vi "STFT - Spectogram.vi"(0 "reference in":refnum<class "SPWB.lvclass">, 5 "error in (no error)":errorcluster, 7 "Ch. Idx":i32, 9 "STFT Parameters":T1={"SVM time segment"={"from [s]"=-1.0, "to [s]"=-1.0, "time increment"=100.0, "time increment units (%)"=enum."%"}, "FFT block size"=1024, "Window type"=1, "dB On (T)"=FALSE, "weighting"=0, "Norm Signal"=FALSE, "time steps"=-1, "STFT Type"=enum."TFA Pkg - STFT", "Color Table"=enum."rainbow"} {"weighting" items=["Linear", "A-weighting", "B-weighting", "C-weighting"]; "Window type" items=["None ", "Hanning", "Hamming", "Blackman-Harris", "Exact Blackman", "Blackman", "Flat Top", "4 Term B-Harris ", "7 Term B-Harris", "Low Sidelobe", "Gaussian"]; "FFT block size" min=1; "SVM time segment"."time increment" format="%.2f"; "SVM time segment"."to [s]" format="%.2f"; "SVM time segment"."from [s]" format="%.2f"}) -> (11 "scale info":variant, 12 "spectrogram UI":dbl[][](array[numeric]), 13 "spectrogram Trends":dbl[][](array[numeric]), 14 "reference out":refnum<class "SPWB.lvclass">, 19 "error out":errorcluster)   [LabVIEW 2020, in "SPWB.lvclass"]
uses:
  SPWB.lvclass
  <vilib>/addons/Time Series Analysis/Series Preprocess.llb/TSA Resampling (Waveform).vi
  <vilib>/addons/Time Frequency Analysis/Spectrogram.llb/TFA STFT Spectrogram (Waveform).vi
  API/GSwFormDSP_class/GSwFormDSP.lvclass
  <vilib>/addons/_Advanced Signal Processing/NI_AdvSigProcTSA.lvlib
  <vilib>/addons/_Advanced Signal Processing/NI_AdvSigProcTFA.lvlib
panel:
  out "Nb Time Steps":i32
  out "Nb Freq.":i32
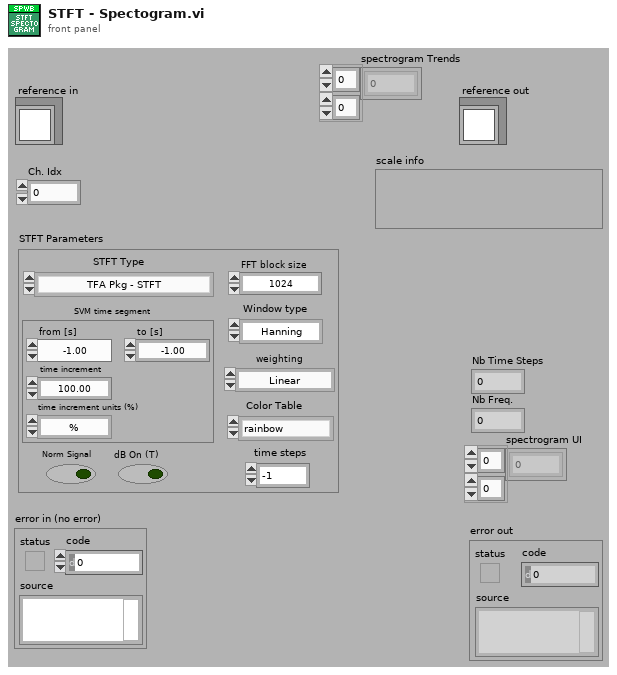
[diagram p1: front panel]
types:
  T1 = cluster{"SVM time segment":cluster{"from [s]":dbl, "to [s]":dbl, "time increment":dbl, "time increment units (%)":enum16{"%", "s", "ms"}}, "FFT block size":i32, "Window type":i32, "dB On (T)":bool, "weighting":u16, "Norm Signal":bool, "time steps":i32, "STFT Type":enum16{"SVM -STFT", "TFA Pkg - STFT"}, "Color Table":enum16{"fire", "rainbow", "grey", "inverse grey", "ice", "original"}}
  T2 = enum16{"None", "To itself", "To the max levels of ALL the signals"}
  T3 = typedef "SPWB.lvclass/ObjectAttributes.ctl" = cluster{"Window Name Index":string, "Data":refnum<class "GSwFormDSP.lvclass">, "Registration":refnum<class "Registration.lvclass">, "TFA User Control Refs ":T4}
  T4 = typedef "SPWB.lvclass/TFA - User Control References.ctl" = cluster{"STFT Graph":refnum<vi>, "Time Section":refnum<vi>, "Frequency Section":refnum<vi>}
  T5 = enum16{"fire", "rainbow", "grey", "inverse grey", "ice", "original"}
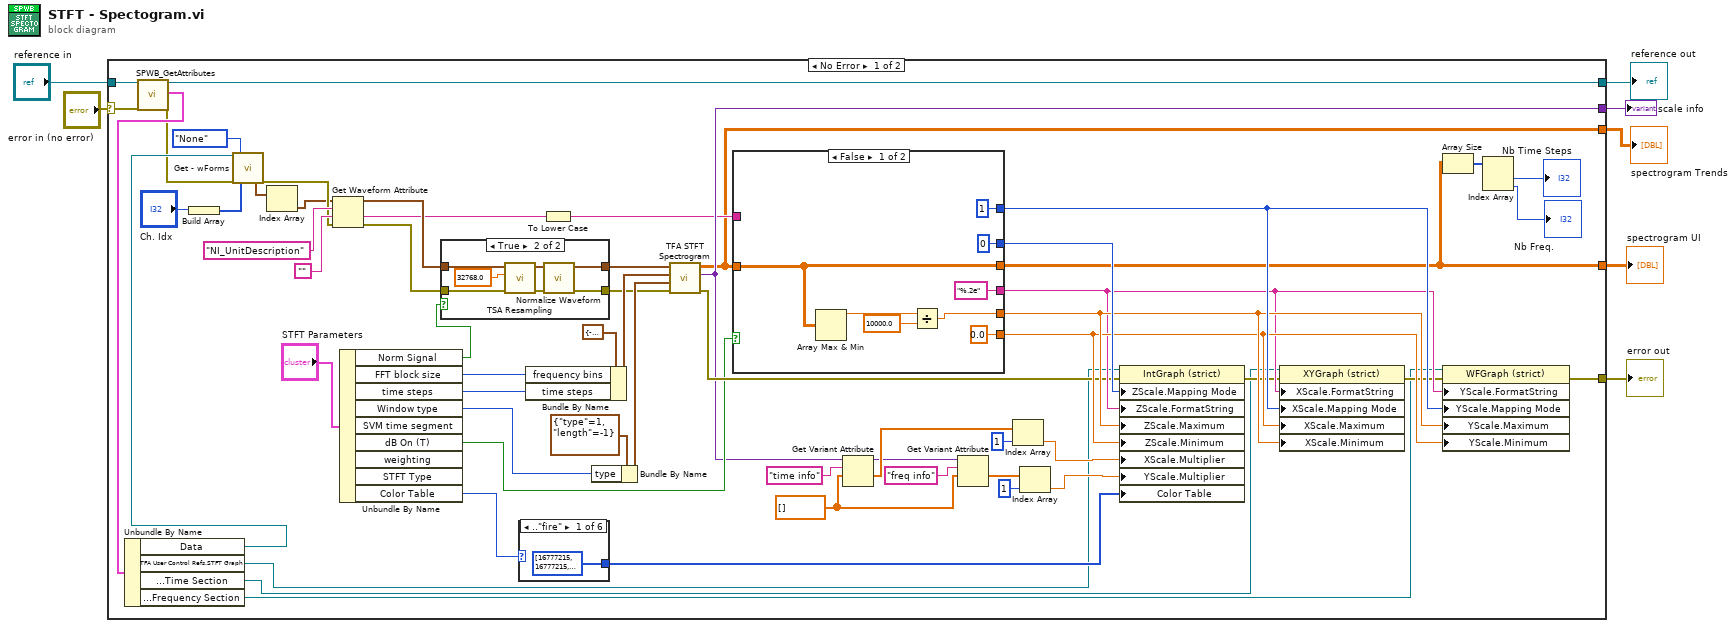
[diagram p0: block diagram]
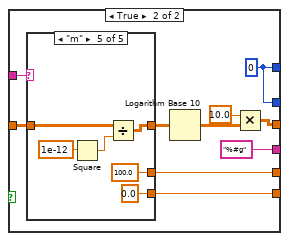
[diagram p2: hidden frame]
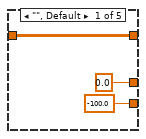
[diagram p3: hidden frame]
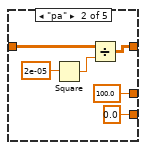
[diagram p4: hidden frame]
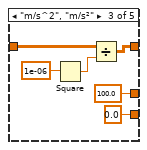
[diagram p5: hidden frame]
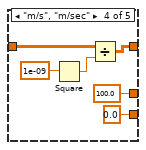
[diagram p6: hidden frame]
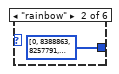
[diagram p7: hidden frame]
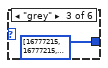
[diagram p8: hidden frame]
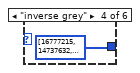
[diagram p9: hidden frame]
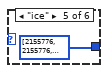
[diagram p10: hidden frame]
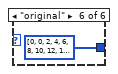
[diagram p11: hidden frame]
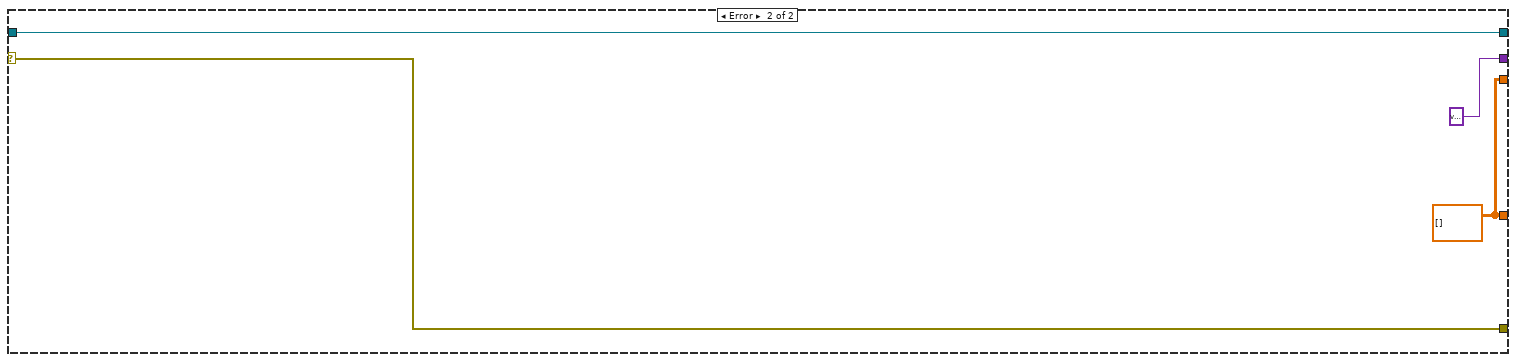
[diagram p13: hidden frame]
diagram:
  n1 = case shown="No Error" "error in (no error)" {
    selector: "error in (no error)" -> [w67 w131]
    tunnel: [w27 w131] -> w6
    tunnel: [w66 w130] -> w4
    tunnel: "reference in" -> [w65 w130]
    tunnel: [w26 w128] -> w3
    tunnel: [w25 variant ("scale info")] -> w2
    tunnel: [w18 w128] -> w1
    frame No Error {
      w58 = dbl[] []
      n2 = call "SPWB_GetAttributes.vi"("reference in"=w65, "error in (no error)"=w67) -> ("reference out"=w66:refnum<class "SPWB.lvclass">, "attributes"=w32:T3, "error out"=w15:errorcluster)  [unwired: 14 in, 1 out]
      n3 = Unbundle By Name(w32) -> ("Data"=w17:refnum<class "GSwFormDSP.lvclass">, "TFA User Control Refs.STFT Graph"=w31:refnum<vi>, "TFA User Control Refs.Time Section"=w30:refnum<vi>, "TFA User Control Refs.Frequency Section"=w29:refnum<vi>)
      n4 = Build Array("Ch. Idx") -> (w13:i32[])
      n5 = call-dynamic "Get - wForms.vi"("reference in"=w17, "error in (no error)"=w15, "Normalization Option"=T2."None", "Indexes (Empty = ALL)"=w13) -> ("wForms"=w11:waveform(dbl)[], "error out"=w12:errorcluster)  [unwired: 12 in, 2 out]
      n6 = Index Array(array=w11) -> (element=w10:waveform(dbl))  [unwired: 1 in]
      n7 = Get Waveform Attribute(4:w12, 5:"", 6:"NI_UnitDescription" ("Att - wform unit"), 7:w10) -> (0:w23:errorcluster, 1:w20:string, 3:w24:waveform(dbl))  [unwired: 1 out]
      n8 = Unbundle By Name("STFT Parameters") -> ("Norm Signal"=w38:bool, "FFT block size"=w9:i32, "time steps"=w8:i32, "Window type"=w34:i32, "dB On (T)"=w33:bool, "Color Table"=w37:T5)  [unwired: 3 out]
      n9 = case shown="True" w38 {
        tunnel: [w120 w127] -> w35
        tunnel: w24 -> [w120 w126]
        tunnel: w23 -> [w119 w122]
        tunnel: [w119 w121] -> w36
        frame False {
        }
        frame True {
          n10 = call-poly <vilib>:"TSA Resampling.vi"("error in (no error)"=w122, "new sampling rate"=32768.0, "Xt"=w126) -> ("error out"=w123:errorcluster, "Xt resampled"=w124:waveform(dbl))  [unwired: 7 in]
          n11 = call <vilib>:"Normalize Waveform.vi"("error in (no error)"=w123, "waveform in"=w124) -> ("error out"=w121:errorcluster, "normalized waveform"=w127:waveform(dbl))  [unwired: 6 in, 2 out]
        }
      }
      n12 = case shown="..\"fire\"" w37 {
        tunnel: [u32[] [16777215, 16777215, 16777215, 16777215, 16777215, 16777215, 16777215, 16777215, 16777212, 16777209, 16777205, 16777202, 16777199, 16777196, 16777193, 16777190, 16777186, 16777183, 16777180, 16777177, 16777174, 16777170, 16777167, 16777164, 16777161, 16777158, 16777154, 16777151, 16777148, 16777145, 16777142, 16777139, 16777135, 16777132, 16777129, 16777126, 16777123, 16777119, 16777116, 16777113, 16777110, 16777107, 16777103, 16777100, 16777097, 16777094, 16777091, 16777088, 16777084, 16777081, 16777078, 16777075, 16777072, 16777068, 16777065, 16777062, 16777059, 16777056, 16777052, 16777049, 16777046, 16777043, 16777040, 16777037, 16777033, 16777030, 16777027, 16777024, 16777021, 16777017, 16777014, 16777011, 16777008, 16777005, 16777001, 16776998, 16776995, 16776992, 16776989, 16776986, 16776982, 16776979, 16776976, 16776973, 16776970, 16776966, 16776963, 16776960, 16776192, 16775424, 16774400, 16773632, 16772864, 16772096, 16771328, 16770560, 16769536, 16768768, 16768000, 16767232, 16766464, 16765440, 16764672, 16763904, 16763136, 16762368, 16761344, 16760576, 16759808, 16759040, 16758272, 16757504, 16756480, 16755712, 16754944, 16754176, 16753408, 16752384, 16751616, 16750848, 16750080, 16749312, 16748288, 16747520, 16746752, 16745984, 16745216, 16744448, 16743424, 16742656, 16741888, 16741120, 16740352, 16739328, 16738560, 16737792, 16737024, 16736256, 16735232, 16734464, 16733696, 16732928, 16732160, 16731392, 16730368, 16729600, 16728832, 16728064, 16727296, 16726272, 16725504, 16724736, 16723968, 16723200, 16722176, 16721408, 16720640, 16719872, 16719104, 16718336, 16717312, 16716544, 16715776, 16715008, 16714240, 16713216, 16712448, 16711680, 16515072, 16318464, 16056320, 15859712, 15663104, 15466496, 15269888, 15073280, 14811136, 14614528, 14417920, 14221312, 14024704, 13762560, 13565952, 13369344, 13172736, 12976128, 12713984, 12517376, 12320768, 12124160, 11927552, 11730944, 11468800, 11272192, 11075584, 10878976, 10682368, 10420224, 10223616, 10027008, 9830400, 9633792, 9371648, 9175040, 8978432, 8781824, 8585216, 8388608, 8126464, 7929856, 7733248, 7536640, 7340032, 7077888, 6881280, 6684672, 6488064, 6291456, 6029312, 5832704, 5636096, 5439488, 5242880, 5046272, 4784128, 4587520, 4390912, 4194304, 3997696, 3735552, 3538944, 3342336, 3145728, 2949120, 2686976, 2490368, 2293760, 2097152, 1900544, 1703936, 1441792, 1245184, 1048576, 851968, 655360, 393216, 196608, 65793, 65793, 65793, 65793, 65793, 65793, 65793, 65793, 0] ("256 fire") u32[] [0, 8388863, 8257791, 8061183, 7930111, 7733503, 7602431, 7405823, 7274751, 7078143, 6947071, 6750463, 6619391, 6422783, 6291711, 6095103, 5964031, 5767423, 5636351, 5439743, 5308671, 5112063, 4980991, 4784383, 4653311, 4456703, 4325631, 4129023, 3932415, 3801343, 3604735, 3473663, 3277055, 3145983, 2949375, 2818303, 2621695, 2490623, 2294015, 2162943, 1966335, 1835263, 1638655, 1507583, 1310975, 1179903, 983295, 852223, 655615, 524543, 327935, 196863, 511, 1791, 3071, 4351, 5631, 6911, 8191, 9471, 10751, 12031, 13311, 14591, 15871, 17151, 18431, 19711, 20991, 22271, 23551, 24831, 26111, 27391, 28671, 29951, 31231, 32511, 33791, 35071, 36351, 37631, 38911, 40191, 41471, 42751, 44031, 45311, 46591, 47871, 49151, 50431, 51711, 52991, 54271, 55551, 56831, 58111, 59391, 60671, 61951, 63231, 64511, 65532, 65527, 65522, 65517, 65512, 65507, 65502, 65497, 65492, 65487, 65482, 65477, 65472, 65467, 65462, 65457, 65452, 65447, 65442, 65437, 65432, 65427, 65422, 65417, 65412, 65407, 65402, 65397, 65392, 65387, 65382, 65377, 65372, 65367, 65362, 65357, 65352, 65347, 65342, 65337, 65332, 65327, 65322, 65317, 65312, 65307, 65302, 65297, 65292, 65287, 65282, 261888, 589568, 917248, 1244928, 1572608, 1900288, 2227968, 2555648, 2883328, 3211008, 3538688, 3866368, 4194048, 4521728, 4849408, 5177088, 5504768, 5832448, 6160128, 6487808, 6815488, 7143168, 7470848, 7798528, 8126208, 8453888, 8781568, 9109248, 9436928, 9764608, 10092288, 10419968, 10747648, 11075328, 11403008, 11730688, 12058368, 12386048, 12713728, 13041408, 13369088, 13696768, 14024448, 14352128, 14679808, 15007488, 15335168, 15662848, 15990528, 16318208, 16645888, 16775936, 16774656, 16773376, 16772096, 16770816, 16769536, 16768256, 16766976, 16765696, 16764416, 16763136, 16761856, 16760576, 16759296, 16758016, 16756736, 16755456, 16754176, 16752896, 16751616, 16750336, 16749056, 16747776, 16746496, 16745216, 16743936, 16742656, 16741376, 16740096, 16738816, 16737536, 16736256, 16734976, 16733696, 16732416, 16731136, 16729856, 16728576, 16727296, 16726016, 16724736, 16723456, 16722176, 16720896, 16719616, 16718336, 16717056, 16715776, 16714496, 16713216, 16711680] ("rainbow") u32[] [16777215, 16777215, 16777215, 16777215, 16777215, 16777215, 16711422, 16711422, 16711422, 16711422, 16711422, 16645629, 16645629, 16645629, 16645629, 16645629, 16645629, 16579836, 16579836, 16579836, 16579836, 16579836, 16514043, 16514043, 16514043, 16514043, 16514043, 16448250, 16448250, 16448250, 16448250, 16448250, 16316664, 16382457, 16382457, 16382457, 16382457, 16316664, 16316664, 16316664, 16316664, 16250871, 16250871, 16250871, 16250871, 16250871, 16185078, 16185078, 16185078, 16185078, 16119285, 16119285, 16119285, 16119285, 16119285, 16053492, 16053492, 16053492, 16053492, 15987699, 15987699, 15987699, 15987699, 15921906, 15987699, 15921906, 15921906, 15856113, 15856113, 15856113, 15856113, 15856113, 15790320, 15790320, 15790320, 15724527, 15724527, 15724527, 15724527, 15658734, 15658734, 15658734, 15658734, 15592941, 15592941, 15592941, 15592941, 15527148, 15527148, 15527148, 15461355, 15461355, 15461355, 15461355, 15395562, 15395562, 15395562, 15395562, 15329769, 15329769, 15329769, 15263976, 15263976, 15263976, 15198183, 15198183, 15198183, 15198183, 15132390, 15132390, 15132390, 15066597, 15066597, 15066597, 15000804, 15000804, 15000804, 14935011, 14935011, 14935011, 14869218, 14869218, 14869218, 14803425, 14803425, 14803425, 14737632, 14737632, 14671839, 14671839, 14671839, 14606046, 14606046, 14606046, 14540253, 14540253, 14540253, 14474460, 14474460, 14408667, 14408667, 14408667, 14342874, 14342874, 14277081, 14277081, 14277081, 14211288, 14211288, 14145495, 14145495, 14079702, 14079702, 14013909, 14013909, 14013909, 13948116, 13948116, 13882323, 13882323, 13816530, 13816530, 13750737, 13750737, 13684944, 13684944, 13619151, 13619151, 13553358, 13553358, 13487565, 13487565, 13421772, 13421772, 13355979, 13290186, 13290186, 13224393, 13224393, 13158600, 13092807, 13092807, 13027014, 13027014, 12961221, 12895428, 12895428, 12829635, 12763842, 12763842, 12698049, 12632256, 12566463, 12566463, 12500670, 12434877, 12434877, 12369084, 12303291, 12237498, 12171705, 12171705, 12105912, 12040119, 11974326, 11908533, 11842740, 11776947, 11711154, 11645361, 11579568, 11513775, 11447982, 11382189, 11316396, 11250603, 11184810, 11119017, 10987431, 10921638, 10855845, 10790052, 10658466, 10592673, 10461087, 10395294, 10329501, 10197915, 10066329, 10000536, 9868950, 9737364, 9605778, 9474192, 9342606, 9211020, 9079434, 8882055, 8750469, 8553090, 8421504, 8224125, 7960953, 7763574, 7500402, 7237230, 6974058, 6645093, 6316128, 5855577, 5395026, 4868682, 4210752, 3289650, 2105376, 0] ("256 log up") u32[] [16777215, 14737632, 13487565, 12632256, 11908533, 11382189, 10921638, 10526880, 10132122, 9803157, 9539985, 9276813, 9013641, 8816262, 8553090, 8421504, 8224125, 8026746, 7895160, 7697781, 7566195, 7434609, 7303023, 7171437, 7039851, 6908265, 6776679, 6710886, 6579300, 6447714, 6381921, 6316128, 6184542, 6118749, 5987163, 5921370, 5855577, 5789784, 5658198, 5592405, 5526612, 5460819, 5395026, 5329233, 5263440, 5197647, 5131854, 5066061, 5000268, 4934475, 4868682, 4802889, 4737096, 4671303, 4605510, 4605510, 4539717, 4473924, 4408131, 4342338, 4342338, 4276545, 4210752, 4210752, 4144959, 4079166, 4013373, 4013373, 3947580, 3881787, 3881787, 3815994, 3750201, 3750201, 3684408, 3684408, 3618615, 3552822, 3552822, 3487029, 3487029, 3421236, 3421236, 3355443, 3289650, 3289650, 3223857, 3223857, 3158064, 3158064, 3092271, 3092271, 3026478, 3026478, 2960685, 2960685, 2894892, 2894892, 2829099, 2829099, 2763306, 2763306, 2763306, 2697513, 2697513, 2631720, 2631720, 2565927, 2565927, 2500134, 2500134, 2500134, 2434341, 2434341, 2368548, 2368548, 2368548, 2302755, 2302755, 2236962, 2236962, 2236962, 2171169, 2171169, 2171169, 2105376, 2105376, 2105376, 2039583, 2039583, 1973790, 1973790, 1973790, 1907997, 1907997, 1907997, 1842204, 1842204, 1842204, 1776411, 1776411, 1776411, 1710618, 1710618, 1710618, 1644825, 1644825, 1644825, 1579032, 1579032, 1579032, 1579032, 1513239, 1513239, 1513239, 1447446, 1447446, 1447446, 1381653, 1381653, 1381653, 1381653, 1315860, 1315860, 1315860, 1315860, 1250067, 1250067, 1250067, 1184274, 1184274, 1184274, 1184274, 1118481, 1118481, 1118481, 1118481, 1052688, 1052688, 1052688, 1052688, 986895, 986895, 986895, 921102, 921102, 921102, 921102, 921102, 855309, 855309, 855309, 855309, 789516, 789516, 789516, 789516, 723723, 723723, 723723, 723723, 657930, 657930, 657930, 657930, 657930, 592137, 592137, 592137, 592137, 526344, 526344, 526344, 526344, 526344, 460551, 460551, 460551, 460551, 460551, 394758, 394758, 394758, 394758, 328965, 328965, 328965, 328965, 328965, 263172, 263172, 263172, 263172, 263172, 197379, 197379, 197379, 197379, 197379, 131586, 131586, 131586, 131586, 131586, 131586, 65793, 65793, 65793, 65793, 65793, 0, 0, 0, 0, 0, 0] ("256 log down") u32[] [2155776, 2155776, 2155776, 2155776, 2155776, 2155776, 2155776, 2155776, 127491, 127491, 127491, 127491, 127491, 127491, 127491, 127491, 522752, 522752, 522752, 522752, 522752, 522752, 522752, 522752, 64018, 64018, 64018, 64018, 64018, 64018, 64018, 64018, 63778, 63778, 63778, 63778, 63778, 63778, 63778, 63778, 63790, 63790, 63790, 63790, 63790, 63790, 63790, 63790, 63797, 63797, 63797, 63797, 63797, 63797, 63797, 63797, 63807, 63807, 63807, 63807, 63807, 63807, 63807, 63807, 64068, 64068, 64068, 64068, 64068, 64068, 64068, 64068, 63828, 63828, 63828, 63828, 63828, 63828, 63828, 63828, 63833, 63833, 63833, 63833, 63833, 63833, 63833, 63833, 63836, 63836, 63836, 63836, 63836, 63836, 63836, 63836, 63836, 63836, 63836, 63836, 63836, 63836, 63836, 63836, 61790, 61790, 61790, 61790, 61790, 61790, 61790, 61790, 58464, 58464, 58464, 58464, 58464, 58464, 58464, 58464, 55387, 55387, 55387, 55387, 55387, 55387, 55387, 55387, 51286, 51286, 51286, 51286, 51286, 51286, 51286, 51286, 47440, 47440, 47440, 47440, 47440, 47440, 47440, 47440, 40284, 40284, 40284, 40284, 40284, 40284, 40284, 40284, 34154, 34154, 34154, 34154, 34154, 34154, 34154, 34154, 28540, 28540, 28540, 28540, 28540, 28540, 28540, 28540, 20113, 20113, 20113, 20113, 20113, 20113, 20113, 20113, 12193, 12193, 12193, 12193, 12193, 12193, 12193, 12193, 12714, 12714, 12714, 12714, 12714, 12714, 12714, 12714, 7351, 7351, 7351, 7351, 7351, 7351, 7351, 7351, 4800, 4800, 4800, 4800, 4800, 4800, 4800, 4800, 195, 195, 195, 195, 195, 195, 195, 195, 189, 189, 189, 189, 189, 189, 189, 189, 183, 183, 183, 183, 183, 183, 183, 183, 175, 175, 175, 175, 175, 175, 175, 175, 164, 164, 164, 164, 164, 164, 164, 164, 155, 155, 155, 155, 155, 155, 155, 155] ("32 ice") u32[] [0, 0, 2, 4, 6, 8, 10, 12, 14, 16, 18, 20, 22, 24, 26, 28, 30, 32, 34, 36, 38, 40, 42, 44, 46, 48, 50, 52, 54, 56, 58, 60, 62, 64, 66, 68, 70, 72, 74, 76, 78, 80, 82, 84, 86, 88, 90, 92, 94, 96, 98, 100, 102, 104, 106, 108, 110, 112, 114, 116, 118, 120, 122, 124, 126, 128, 130, 132, 134, 136, 138, 140, 142, 144, 146, 148, 150, 152, 154, 156, 158, 160, 162, 164, 166, 168, 170, 172, 174, 176, 178, 180, 182, 184, 186, 188, 190, 192, 194, 196, 198, 200, 202, 204, 206, 208, 210, 212, 214, 216, 218, 220, 222, 224, 226, 228, 230, 232, 234, 236, 238, 240, 242, 244, 246, 248, 250, 252, 255, 131839, 263423, 395007, 526591, 658175, 789759, 921343, 1052927, 1184511, 1316095, 1447679, 1579263, 1710847, 1842431, 1974015, 2105599, 2237183, 2368767, 2500351, 2631935, 2763519, 2895103, 3026687, 3158271, 3289855, 3421439, 3553023, 3684607, 3816191, 3947775, 4079359, 4210943, 4342527, 4474111, 4605695, 4737279, 4868863, 5000447, 5132031, 5263615, 5395199, 5526783, 5658367, 5789951, 5921535, 6053119, 6184703, 6316287, 6447871, 6579455, 6711039, 6842623, 6974207, 7105791, 7237375, 7368959, 7500543, 7632127, 7763711, 7895295, 8026879, 8158463, 8290047, 8421631, 8553215, 8684799, 8816383, 8947967, 9079551, 9211135, 9342719, 9474303, 9605887, 9737471, 9869055, 10000639, 10132223, 10263807, 10395391, 10526975, 10658559, 10790143, 10921727, 11053311, 11184895, 11316479, 11448063, 11579647, 11711231, 11842815, 11974399, 12105983, 12237567, 12369151, 12500735, 12632319, 12763903, 12895487, 13027071, 13158655, 13290239, 13421823, 13553407, 13684991, 13816575, 13948159, 14079743, 14211327, 14342911, 14474495, 14606079, 14737663, 14869247, 15000831, 15132415, 15263999, 15395583, 15527167, 15658751, 15790335, 15921919, 16053503, 16185087, 16316671, 16448255, 16579839, 16777215] ("original")] -> w42
        frame .."fire" {
        }
        frame "rainbow" {
        }
        frame "grey" {
        }
        frame "inverse grey" {
        }
        frame "ice" {
        }
        frame "original" {
        }
      }
      n13 = Bundle By Name(cluster=cluster{"time steps":i32, "frequency bins":i32} {"time steps"=-1, "frequency bins"=512} ("time-frequency sampling info"), "frequency bins"=w9, "time steps"=w8) -> (w54:cluster{"time steps":i32, "frequency bins":i32})
      n14 = To Lower Case(string=w20) -> (all lower case string=w19:string)
      n15 = Bundle By Name(cluster=cluster{"type":i32, "length":i32} {"type"=1, "length"=-1} ("window info"), "type"=w34) -> (w63:cluster{"type":i32, "length":i32})
      n16 = call-poly <vilib>:"TFA STFT Spectrogram.vi"("error in (no error)"=w36, "window info"=w63, "time-frequency sampling info"=w54, "signal"=w35) -> ("error out"=w39:errorcluster, "scale info"=w25:variant, "spectrogram"=w18:dbl[][])  [unwired: 5 in]
      n17 = case shown="False" w33 {
        tunnel: w18 -> [w74 w79]
        tunnel: [w74 w83] -> w26
        tunnel: [w71 w78] -> w47
        tunnel: [0.0 w77] -> w46
        tunnel: ["%.2e" "%#g"] -> w45
        tunnel: [u8 1 ("X Scale.Mapping Mode") w82] -> w48
        tunnel: [u8 0 ("X Scale.Mapping Mode") w82] -> w49
        tunnel: w19 -> [_ w81]
        frame False {
          n18 = Array Max & Min(array=w74) -> (max value=w72:dbl)  [unwired: 3 out]
          n19 = Divide(x=w72, y=10000.0) -> (x/y=w71:dbl)
        }
        frame True {
          w82 = u8 0 ("X Scale.Mapping Mode")
          n20 = case shown="\"m\"" w81 {
            tunnel: [w88 w93 w99 w105 w111] -> w80
            tunnel: w79 -> [w88 w94 w100 w106 w112]
            tunnel: [0.0 100.0 100.0 100.0 100.0] -> w78
            tunnel: [-100.0 0.0 0.0 0.0 0.0] -> w77
            frame "", Default {
            }
            frame "pa" {
              n21 = Square(x=2e-05) -> (x^2=w91:dbl)
              n22 = Divide(x=w94, y=w91) -> (x/y=w93:dbl[][])
            }
            frame "m/s^2", "m/s²" {
              n23 = Square(x=1e-06) -> (x^2=w98:dbl)
              n24 = Divide(x=w100, y=w98) -> (x/y=w99:dbl[][])
            }
            frame "m/s", "m/sec" {
              n25 = Square(x=1e-09) -> (x^2=w104:dbl)
              n26 = Divide(x=w106, y=w104) -> (x/y=w105:dbl[][])
            }
            frame "m" {
              n27 = Square(x=1e-12) -> (x^2=w110:dbl)
              n28 = Divide(x=w112, y=w110) -> (x/y=w111:dbl[][])
            }
          }
          n29 = Logarithm Base 10(1:w80) -> (0:w85:dbl[][])
          n30 = Multiply(x=10.0, y=w85) -> (x*y=w83:dbl[][])
        }
      }
      n31 = Get Variant Attribute(Variant=w25, name="time info", default value (empty Variant)=w58) -> (duplicate Variant=w59:variant, value=w61:dbl[])  [unwired: 1 in, 2 out]
      n32 = Get Variant Attribute(Variant=w59, name="freq info", default value (empty Variant)=w58) -> (value=w64:dbl[])  [unwired: 1 in, 3 out]
      n33 = Index Array(array=w61, index=1) -> (element=w40:dbl)
      n34 = Index Array(array=w64, index=1) -> (element=w41:dbl)
      n35 = property class="IntGraph (strict)"(reference=w31, error in=w39, "ZScale.Mapping Mode"=w49, "ZScale.FormatString"=w45, "ZScale.Maximum"=w47, "ZScale.Minimum"=w46, "XScale.Multiplier"=w40, "YScale.Multiplier"=w41, "Color Table"=w42) -> (error out=w43:errorcluster)  [unwired: 1 out]
      n36 = property class="XYGraph (strict)"(reference=w30, error in=w43, "XScale.FormatString"=w45, "XScale.Mapping Mode"=w48, "XScale.Maximum"=w46, "XScale.Minimum"=w47) -> (error out=w44:errorcluster)  [unwired: 1 out]
      n37 = Array Size(array=w26) -> (size(s)=w28:i32[])
      n38 = property class="WFGraph (strict)"(reference=w29, error in=w44, "YScale.FormatString"=w45, "YScale.Mapping Mode"=w48, "YScale.Maximum"=w47, "YScale.Minimum"=w46) -> (error out=w27:errorcluster)  [unwired: 1 out]
      n39 = Index Array(array=w28) -> (element #1=→"Nb Time Steps":i32, element #2=→"Nb Freq.":i32)  [unwired: 2 in]
    }
    frame Error {
      w128 = dbl[][] [] ("spectrogram")
    }
  }
  "error out" <- w6
  "reference out" <- w4
  "spectrogram UI" <- w3
  "scale info" <- w2
  "spectrogram Trends" <- w1
